vi "Exclude Paths.vi"(8 "error in (no error)":errorcluster, 11 "Search in":refnum<class "Search.lvclass">) -> (0 "error out":errorcluster, 2 "Exclude Paths":path[](array[path]), 3 "Search out":refnum<class "Search.lvclass">)   [LabVIEW 2016, in "Better Search.lvlib" / "Search.lvclass"]
uses:
  Search.lvclass
  Better Search.lvlib
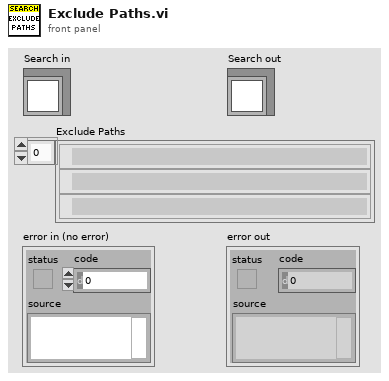
[diagram p1: front panel]
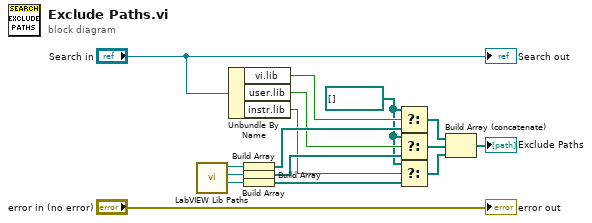
[diagram p0: block diagram]
diagram:
  w5 = path[] [] ("t")
  n1 = call "LabVIEW Lib Paths.vi"() -> ("instr.lib"=w15:path, "user.lib"=w14:path, "vi.lib"=w13:path)  [unwired: 9 in]
  n2 = Unbundle By Name("Search in") -> ("vi.lib"=w6:bool, "user.lib"=w7:bool, "instr.lib"=w8:bool)
  n3 = Build Array(w13) -> (w10:path[])
  n4 = Build Array(w14) -> (w11:path[])
  n5 = Build Array(w15) -> (w12:path[])
  n6 = Select(t=w5, s=w6, f=w10) -> (s? t:f=w3:path[])
  n7 = Select(t=w5, s=w7, f=w11) -> (s? t:f=w4:path[])
  n8 = Select(t=w5, s=w8, f=w12) -> (s? t:f=w2:path[])
  n9 = Build Array (concatenate)(w3, w4, w2) -> (→"Exclude Paths":path[])
  "error out" <- "error in (no error)"
  "Search out" <- "Search in"
